vi "St Dev Threshold Testing.vi"() -> ()   [LabVIEW 2018]
uses:
  <vilib>/DAQmx/read.llb/DAQmx Read (Analog Wfm 1Chan 1Samp).vi
  <vilib>/DAQmx/create/channels.llb/DAQmx Create Channel (AI-Voltage-Basic).vi
  <vilib>/DAQmx/miscellaneous.llb/DAQmx Fill In Error Info.vi
  <vilib>/Waveform/WDTOps.llb/WDT Append Waveforms DBL.vi
  <vilib>/measure/mamon.llb/Limit Testing Time.vi
  <vilib>/measure/NI_MAPro.lvlib
  <vilib>/ptbypt/NI_PtbyPt.lvlib
panel:
  in  "sample length":i32=100
  in  "# of sigmas":dbl
  out "Limit Test":waveform(dbl)[](graph)
  out "st deviation":dbl(graph)
  out "mean":dbl(graph)
  out "readings":waveform(dbl)(graph)
  in  "stop":bool
  in  "Diode":tag
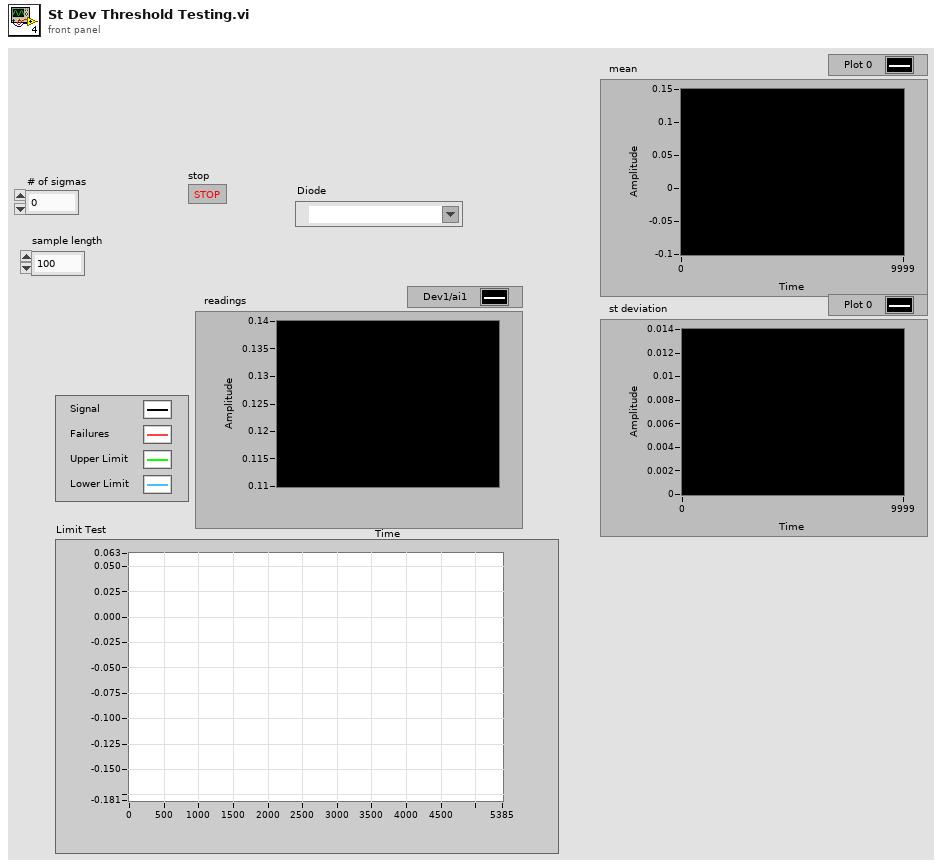
[diagram p1: front panel]
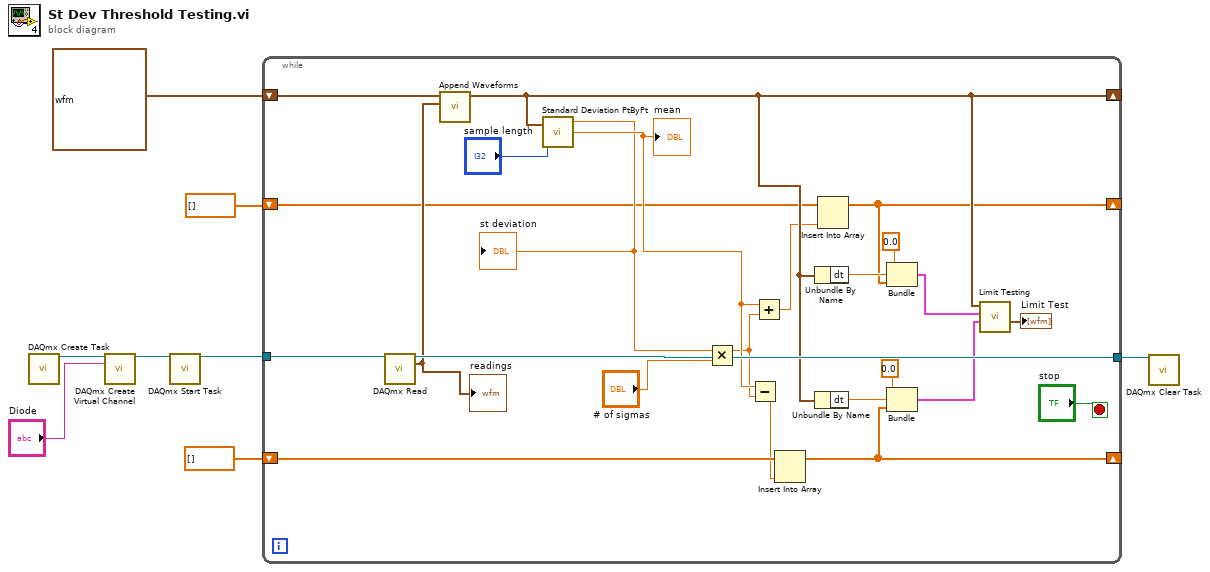
[diagram p0: block diagram]
diagram:
  n1 = call <vilib>:"DAQmx Create Task.vi"() -> ("task out"=w8:refnum<k21>)  [unwired: 14 in, 1 out]
  n2 = call-poly <vilib>:"DAQmx Create Virtual Channel.vi"("task in"=w8, "physical channels"="Diode") -> ("task out"=w7:refnum<k21>)  [unwired: 12 in, 1 out]
  n3 = call <vilib>:"DAQmx Start Task.vi"("task/channels in"=w7) -> ("task out"=w5:refnum<k21>)  [unwired: 13 in, 1 out]
  n4 = while {
    tunnel: w5 -> [w32]
    shift-right: [w22] -> _
    shift-left: waveform(dbl) {"t0"=timestamp(0 s since 1904-01-01), "dt"=1.0, "Y"=[]} ("Waveform") -> [w29]
    tunnel: [w31] -> w4
    shift-right: [w15] -> _
    shift-left: dbl[] [] -> [w17]
    shift-right: [w11] -> _
    shift-left: dbl[] [] -> [w13]
    stop <- "stop" stop-if-true
    n5 = call-poly <vilib>:"DAQmx Read.vi"("task/channels in"=w32) -> ("task out"=w31:refnum<k21>, "data"=w28:waveform(dbl))  [unwired: 12 in, 1 out]
    "readings" <- w28
    n6 = call-poly <vilib>:"Append Waveforms.vi"("waveform B"=w28, "waveform A"=w29) -> ("waveform out"=w22:waveform(dbl))  [unwired: 8 in, 1 out]
    n7 = call <vilib>:"Standard Deviation PtByPt.vi"("x"=w22, "sample length"="sample length") -> ("standard deviation"=w20:dbl, "mean"=w21:dbl)  [unwired: 1 in, 1 out]
    "mean" <- w21
    "st deviation" <- w20
    n8 = Multiply(x=w20, y="# of sigmas") -> (x*y=w19:dbl)
    n9 = Subtract(x=w21, y=w19) -> (x-y=w12:dbl)
    n10 = Add(x=w21, y=w19) -> (x+y=w14:dbl)
    n11 = Insert Into Array(array=w13, new element=w12) -> (w11:dbl[])  [unwired: 1 in]
    n12 = Unbundle By Name(w22) -> ("dt"=w26:dbl)
    n13 = Unbundle By Name(w22) -> ("dt"=w24:dbl)
    n14 = Insert Into Array(array=w17, new element=w14) -> (w15:dbl[])  [unwired: 1 in]
    n15 = Bundle(0.0, "dt"=w26, w15) -> (w16:cluster{dbl, "dt":dbl, dbl[]})  [unwired: 1 in]
    n16 = Bundle(0.0, "dt"=w24, w11) -> (w10:cluster{dbl, "dt":dbl, dbl[]})  [unwired: 1 in]
    n17 = call-poly <vilib>:"Limit Testing.vi"("lower limit"=w10, "upper limit"=w16, "signal in"=w22) -> ("output values"=→"Limit Test":waveform(dbl)[])  [unwired: 3 in, 5 out]
  }
  n18 = call <vilib>:"DAQmx Clear Task.vi"("task in"=w4) -> ()  [unwired: 14 in, 1 out]
